vi "测试报告摘要.vi"(8 "打印?":bool, 11 "报告时间":timestamp) -> ()   [LabVIEW 2010]
uses:
  <vilib>/Utility/NIReport.llb/NI_report.lvclass
  <vilib>/Utility/NIReport.llb/Append Report Text (str wrap).vi
  全局量/试验配置信息.vi
  全局量/自动测试结果.vi
  <vilib>/addons/_office/NI_ReportGenerationToolkit.lvlib
  <vilib>/addons/_office/word.llb/Word Easy Table (str).vi
panel:
  out "XY图":cluster{"Y":dbl[], "Y":dbl[]}[](graph)
  # "T：打印\nF：保存"
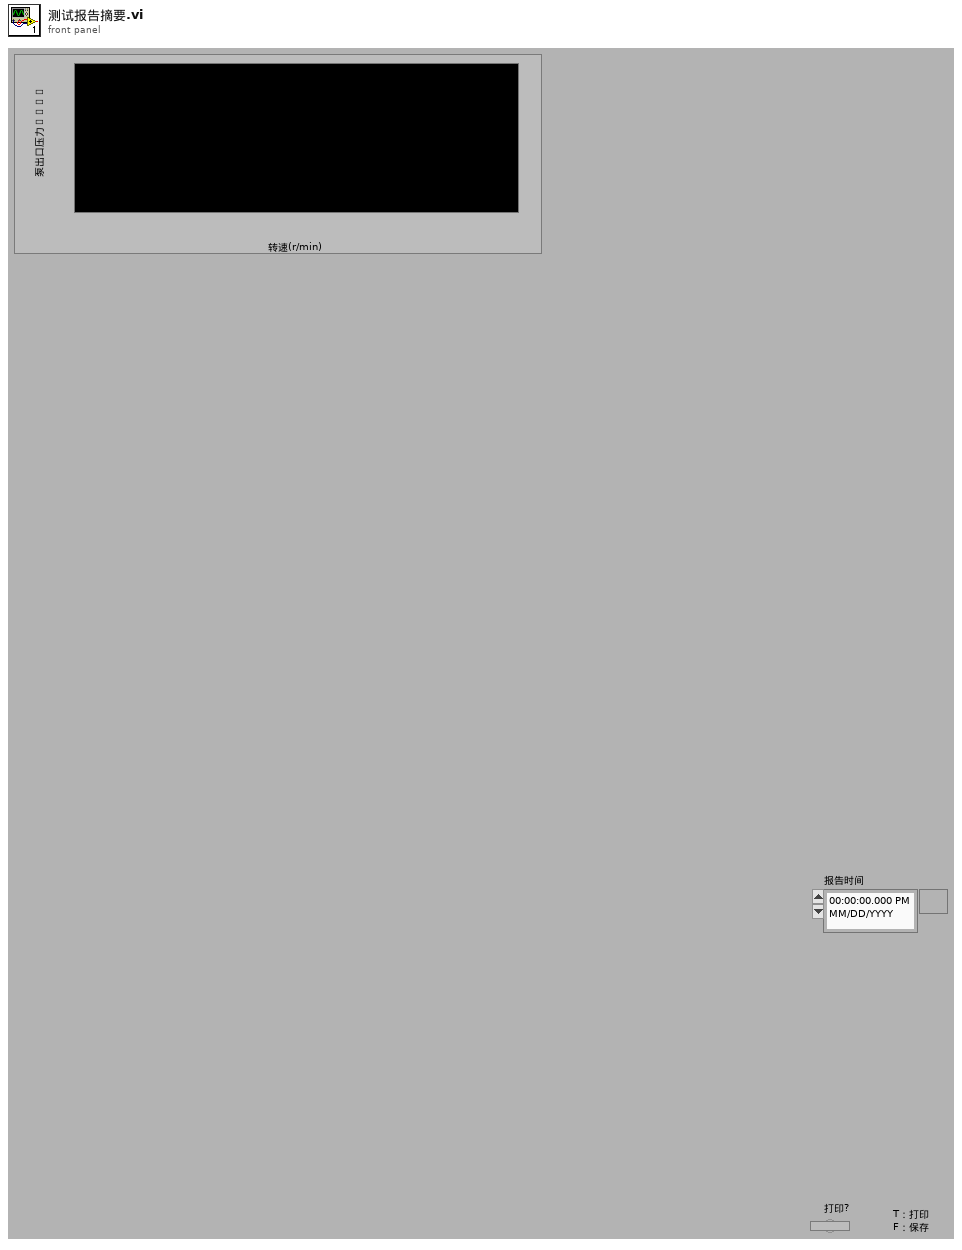
[diagram p1: front panel]
types:
  T1 = cluster{"position (Excel)":cluster{"row":i32, "column":i32}, "name (Excel)":string, "bookmark (Word)":string}
  T2 = enum16{"maximized", "minimized", "normal", "no change"}
  T3 = enum16{"Standard Report", "HTML", "Word", "Excel"}
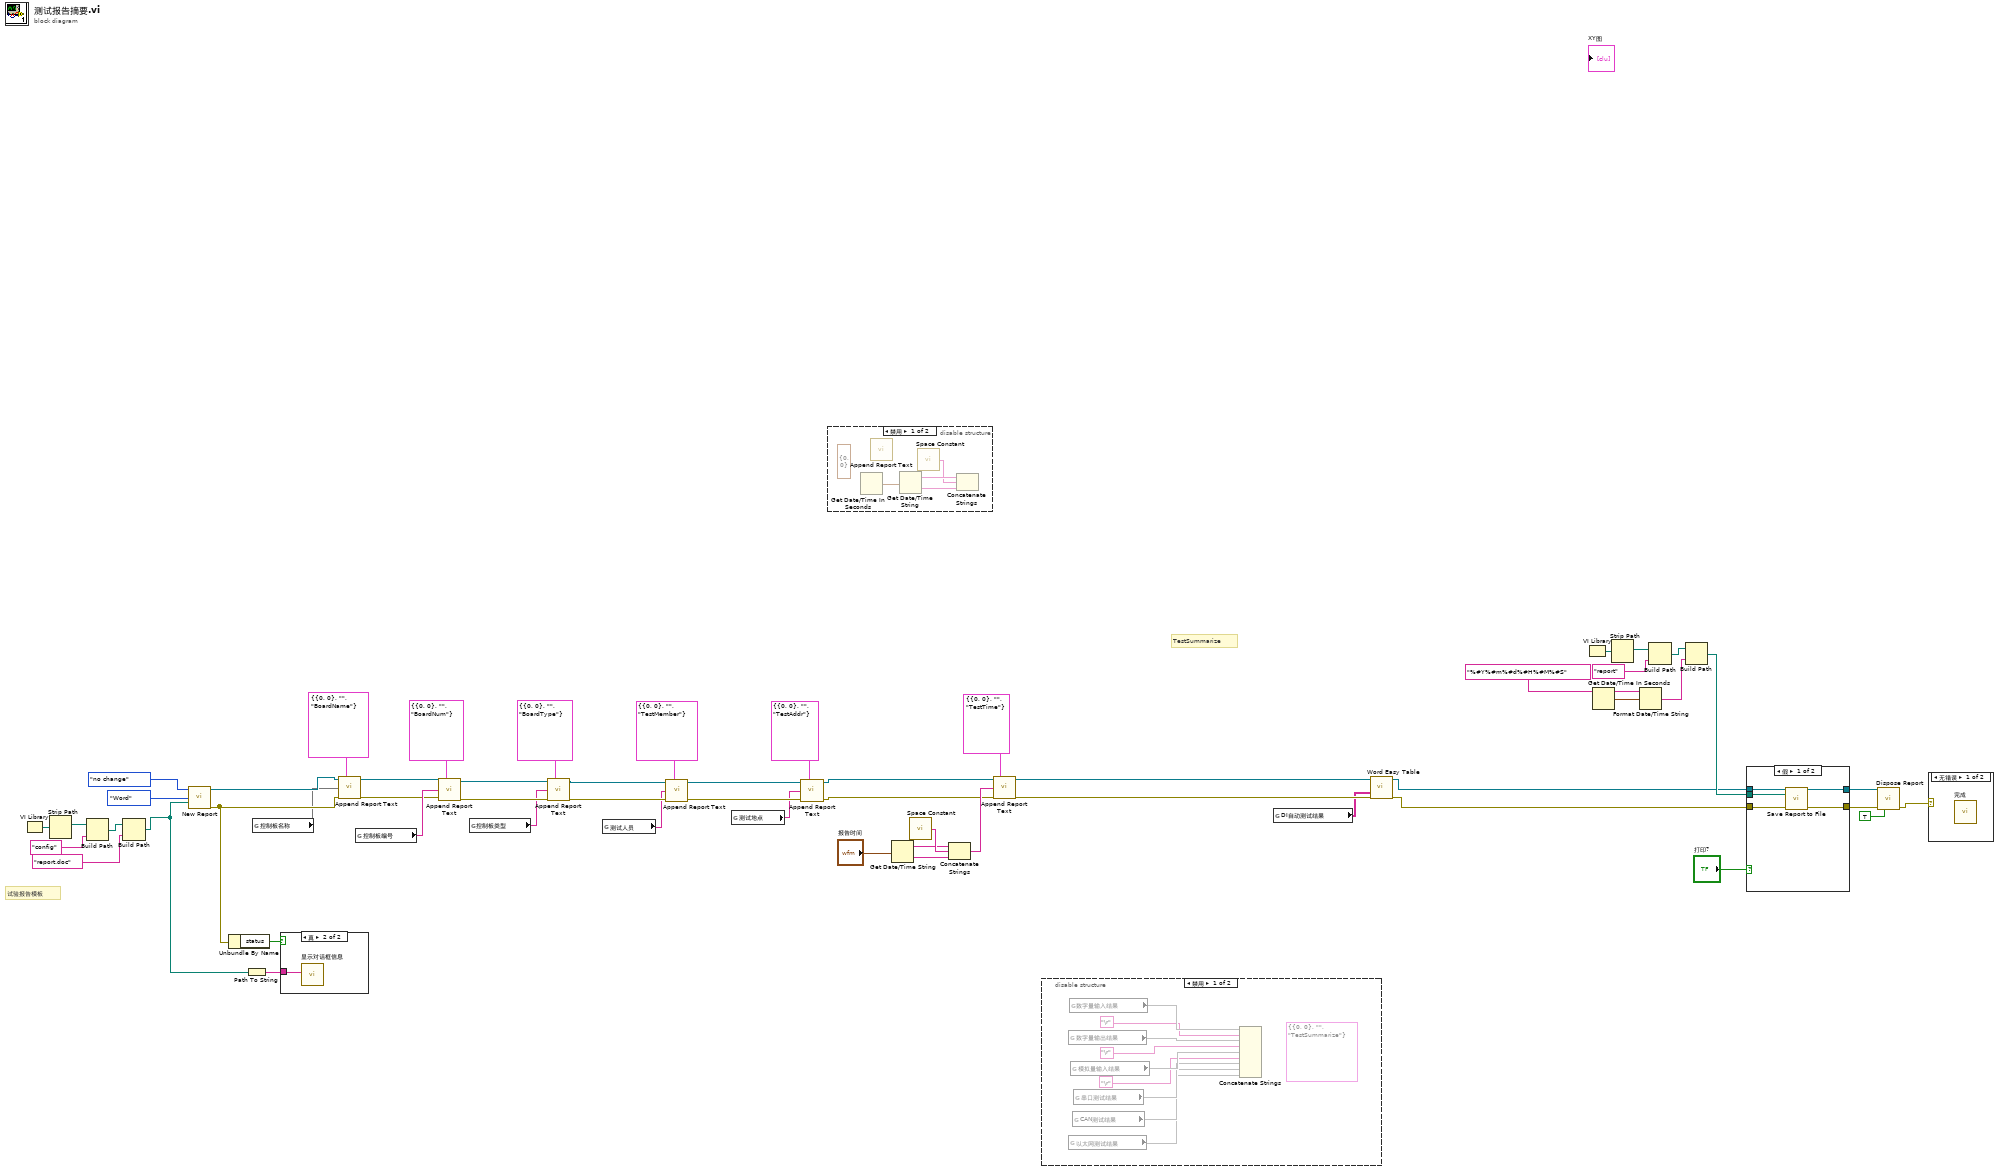
[diagram p0: block diagram]
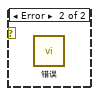
[diagram p3: hidden frame]
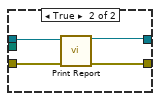
[diagram p4: hidden frame]
diagram:
  # "TestSummarize"
  # "试验报告模板"
  n1 = VI Library() -> (path=w51:path)
  n2 = Strip Path(path=w51) -> (stripped path=w48:path)  [unwired: 1 out]
  n3 = Build Path(base path=w48, name or relative path="config") -> (appended path=w50:path)
  n4 = Build Path(base path=w50, name or relative path="report.doc") -> (appended path=w54:path)
  n5 = call <vilib>:"New Report.vi"("window state (normal)"=T2."no change", "report type"=T3."Word", "template (empty)"=w54) -> ("report out"=w45:refnum<class "NI_report.lvclass">, "error out"=w44:errorcluster)  [unwired: 11 in]
  n6 = Unbundle By Name(w44) -> ("status"=w56:bool)
  n7 = Path To String(path=w54) -> (string=w55:string)
  n8 = global read "试验配置信息.vi" "控制板名称"() -> (w7)
  n9 = case shown="真" w56 {
    tunnel: w55 -> [_ w57]
    frame False {
    }
    frame True {
      n10 = call "显示对话框信息"("Message"=w57) -> ()  [unwired: 9 in, 2 out]
    }
  }
  n11 = call-poly <vilib>:"Append Report Text.vi"("report in"=w45, "MS Office parameters"=T1 {"position (Excel)"={"row"=0, "column"=0}, "name (Excel)"="", "bookmark (Word)"="BoardName"}, "text"=w7, "error in (no error)"=w44) -> ("report out"=w22:refnum<class "NI_report.lvclass">, "error out"=w21:errorcluster)  [unwired: 8 in, 2 out]
  n12 = global read "试验配置信息.vi" "控制板编号"() -> (w23:string)
  n13 = call-poly <vilib>:"Append Report Text.vi"("report in"=w22, "MS Office parameters"=T1 {"position (Excel)"={"row"=0, "column"=0}, "name (Excel)"="", "bookmark (Word)"="BoardNum"}, "text"=w23, "error in (no error)"=w21) -> ("report out"=w35:refnum<class "NI_report.lvclass">, "error out"=w34:errorcluster)  [unwired: 8 in, 2 out]
  n14 = global read "试验配置信息.vi" "控制板类型"() -> (w20:string)
  n15 = call-poly <vilib>:"Append Report Text.vi"("report in"=w35, "MS Office parameters"=T1 {"position (Excel)"={"row"=0, "column"=0}, "name (Excel)"="", "bookmark (Word)"="BoardType"}, "text"=w20, "error in (no error)"=w34) -> ("report out"=w32:refnum<class "NI_report.lvclass">, "error out"=w31:errorcluster)  [unwired: 8 in, 2 out]
  n16 = global read "试验配置信息.vi" "测试人员"() -> (w25:string)
  n17 = call-poly <vilib>:"Append Report Text.vi"("report in"=w32, "MS Office parameters"=T1 {"position (Excel)"={"row"=0, "column"=0}, "name (Excel)"="", "bookmark (Word)"="TestMember"}, "text"=w25, "error in (no error)"=w31) -> ("report out"=w29:refnum<class "NI_report.lvclass">, "error out"=w28:errorcluster)  [unwired: 8 in, 2 out]
  n18 = global read "试验配置信息.vi" "测试地点"() -> (w24:string)
  n19 = call-poly <vilib>:"Append Report Text.vi"("report in"=w29, "MS Office parameters"=T1 {"position (Excel)"={"row"=0, "column"=0}, "name (Excel)"="", "bookmark (Word)"="TestAddr"}, "text"=w24, "error in (no error)"=w28) -> ("report out"=w27:refnum<class "NI_report.lvclass">, "error out"=w26:errorcluster)  [unwired: 8 in, 2 out]
  n20 = disable-structure shown="禁用" {
    frame Disabled {
      (unwired) cluster{"row":i32, "column":i32} {"row"=0, "column"=0} ("position (excel)")
      n21 = Get Date/Time In Seconds() -> (seconds since 1Jan1904=w61:timestamp)
      n22 = call-poly <vilib>:"Append Report Text.vi"() -> ()  [unwired: 12 in, 4 out]
      n23 = Get Date/Time String(seconds (now)=w61) -> (date string=w60:string, time string=w59:string)  [unwired: 2 in]
      n24 = call <vilib>:"Space Constant.vi"() -> ("String"=w58:string)
      n25 = Concatenate Strings(w60, w58, w59) -> ()  [unwired: 1 out]
    }
    frame Enabled {
    }
  }
  n26 = Get Date/Time String(seconds (now)="报告时间") -> (date string=w40:string, time string=w41:string)  [unwired: 2 in]
  n27 = call <vilib>:"Space Constant.vi"() -> ("String"=w42:string)
  n28 = Concatenate Strings(w40, w42, w41) -> (w39:string)
  n29 = call-poly <vilib>:"Append Report Text.vi"("report in"=w27, "MS Office parameters"=T1 {"position (Excel)"={"row"=0, "column"=0}, "name (Excel)"="", "bookmark (Word)"="TestTime"}, "text"=w39, "error in (no error)"=w26) -> ("report out"=w5:refnum<class "NI_report.lvclass">, "error out"=w4:errorcluster)  [unwired: 8 in, 2 out]
  n30 = disable-structure shown="禁用" {
    frame Disabled {
      (unwired) T1 {"position (Excel)"={"row"=0, "column"=0}, "name (Excel)"="", "bookmark (Word)"="TestSummarize"} ("MS Office parameters")
      n31 = global read "自动测试结果.vi" "数字量输出结果"() -> (w68)
      n32 = global read "自动测试结果.vi" "以太网测试结果"() -> (w62)
      n33 = global read "自动测试结果.vi" "数字量输入结果"() -> (w70)
      n34 = global read "自动测试结果.vi" "模拟量输入结果"() -> (w66)
      n35 = global read "自动测试结果.vi" "CAN测试结果"() -> (w63)
      n36 = global read "自动测试结果.vi" "串口测试结果"() -> (w64)
      n37 = Concatenate Strings(w70, "\r", w68, "\r", w66, "\r", w64, w63, w62) -> ()  [unwired: 1 out]
    }
    frame Enabled {
    }
  }
  n38 = global read "自动测试结果.vi" "DI自动测试结果"() -> (w1:string[][])
  n39 = call-poly <vilib>:"Word Easy Table.vi"("report in"=w5, "data"=w1, "error in (no error)"=w4) -> ("report out"=w3:refnum<class "NI_report.lvclass">, "error out"=w2:errorcluster)  [unwired: 10 in, 1 out]
  n40 = VI Library() -> (path=w15:path)
  n41 = Get Date/Time In Seconds() -> (seconds since 1Jan1904=w14:timestamp)
  n42 = Strip Path(path=w15) -> (stripped path=w18:path)  [unwired: 1 out]
  n43 = Format Date/Time String(time format string (%c)="%#Y%#m%#d%#H%#M%#S" ("时间格式字符串(%c)"), seconds (now)=w14) -> (date/time string=w8:string)  [unwired: 1 in]
  n44 = Build Path(base path=w18, name or relative path="report") -> (appended path=w16:path)
  n45 = Build Path(base path=w16, name or relative path=w8) -> (appended path=w9:path)
  n46 = case shown="假" "打印?" {
    tunnel: w3 -> [w75 w79]
    tunnel: w2 -> [w74 w78]
    tunnel: [w73 w77] -> w12
    tunnel: [w72 w76] -> w11
    tunnel: w9 -> [w71 _]
    frame False {
      n47 = call-dynamic "Save Report to File.vi"("report in"=w75, "report file path"=w71, "error in (no error)"=w74) -> ("report out"=w73:refnum<class "NI_report.lvclass">, "error out"=w72:errorcluster)  [unwired: 11 in]
    }
    frame True {
      n48 = call-dynamic "Print Report.vi"("report in"=w79, "error in (no error)"=w78) -> ("report out"=w77:refnum<class "NI_report.lvclass">, "error out"=w76:errorcluster)  [unwired: 12 in]
    }
  }
  n49 = call-dynamic "Dispose Report.vi"("report in"=w12, "error in (no error)"=w11, "close report? (T)"=TRUE) -> ("error out"=w6:errorcluster)  [unwired: 12 in]
  n50 = case shown="无错误" w6 {
    frame No Error {
      n51 = call "完成"() -> ()  [unwired: 10 in, 2 out]
    }
    frame Error {
      n52 = call "错误"() -> ()  [unwired: 10 in, 2 out]
    }
  }
